vi "internalResistance.vi"(8 "Stop":bool, 9 "loaded circuit voltage":dbl=1.2 format="%#_13g", 10 "open circuit voltage":dbl) -> (1 "Internal resistance":dbl format="%#_gohm")   [LabVIEW 2021]
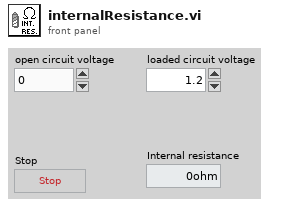
[diagram p1: front panel]
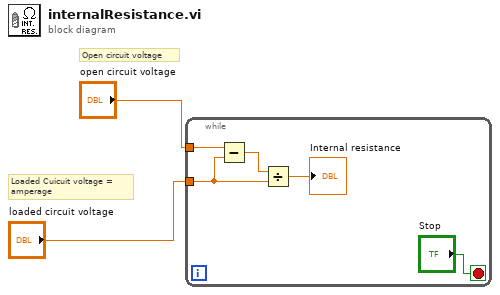
[diagram p0: block diagram]
diagram:
  # "Loaded Cuicuit voltage = \namperage"
  # "Open circuit voltage"
  n1 = while {
    tunnel: "open circuit voltage" -> [w6]
    tunnel: "loaded circuit voltage" -> [w4]
    stop <- "Stop" stop-if-true
    n2 = Subtract(x=w6, y=w4) -> (x-y=w5:dbl)
    n3 = Divide(x=w5, y=w4) -> (x/y=→"Internal resistance":dbl)
  }
